vi "Error Message Window.vi"(11 "eMsg":string) -> ()   [LabVIEW 2012]
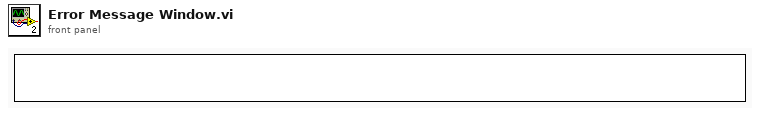
[diagram p1: front panel]
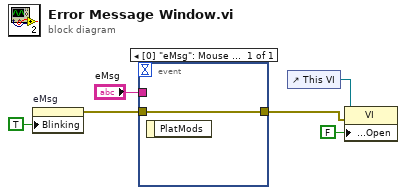
[diagram p0: block diagram]
diagram:
  n1 = property on="eMsg" class="Str"("Blinking"=TRUE) -> (error out=w4:errorcluster)  [unwired: 2 in, 1 out]
  n2 = event shown="[0] \"eMsg\": Mouse Down" {
    selector: _ -> [_]
    dyn-events: _ -> [_]
    timeout: _ -> [_]
    tunnel: "eMsg" -> [_]
    tunnel: w4 -> [w7]
    tunnel: [w7] -> w1
    event "eMsg": Mouse Down {
      n3 = event-data() -> ()  [unwired: 1 in, 1 out]
    }
  }
  n4 = control-ref of="This VI"() -> (w3:refnum<vi>)
  n5 = property class="VI"(reference=w3, error in=w1, "Front Panel.Open"=FALSE ("Front Panel Window:Open")) -> ()  [unwired: 2 out]
